vi "Write Array refnum.vi"(8 "error in (no error)":errorcluster, 10 "Array refnum":refnum<vi>, 11 "Generic Prompt in":refnum<class "Generic Prompt.lvclass">) -> (0 "error out":errorcluster, 3 "Generic Prompt out":refnum<class "Generic Prompt.lvclass">)   [LabVIEW 2014, in "Generic Prompt.lvlib" / "Generic Prompt.lvclass"]
uses:
  Generic Prompt.lvclass
  Subpanel Insertion/Subpanel Inserter.lvclass
  Generic Prompt.lvclass/Generic Prompt.ctl
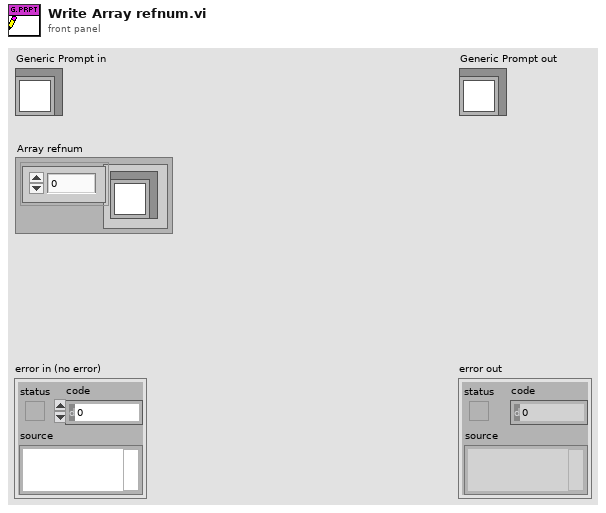
[diagram p1: front panel]
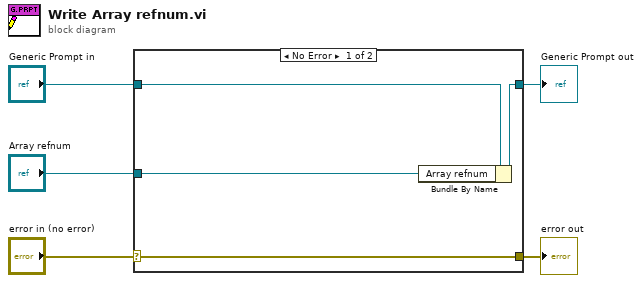
[diagram p0: block diagram]
diagram:
  n1 = case shown="No Error" "error in (no error)" {
    selector: "error in (no error)" -> [w9 w10]
    tunnel: [w9 w10] -> w4
    tunnel: [w7 w11] -> w2
    tunnel: "Generic Prompt in" -> [w8 w11]
    tunnel: "Array refnum" -> [w6 _]
    frame No Error {
      n2 = Bundle By Name(cluster=w8, "Array refnum"=w6) -> (w7:refnum<class "Generic Prompt.lvclass">)
    }
    frame Error {
    }
  }
  "error out" <- w4
  "Generic Prompt out" <- w2
